vi "Clear Handle Map.vi"(8 "error in (no error)":errorcluster, 11 "TwinCAT ADS in":refnum<class "TwinCAT ADS.lvclass">) -> (0 "error out":errorcluster, 3 "TwinCAT ADS out":refnum<class "TwinCAT ADS.lvclass">)   [LabVIEW 2018, in "TwinCAT ADS.lvclass"]
uses:
  TwinCAT ADS.lvclass
  TwinCAT ADS.lvclass/TwinCAT ADS.ctl
panel:
  out "[Symbol Name]":string[](array[string])
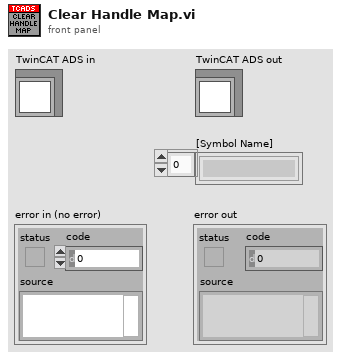
[diagram p1: front panel]
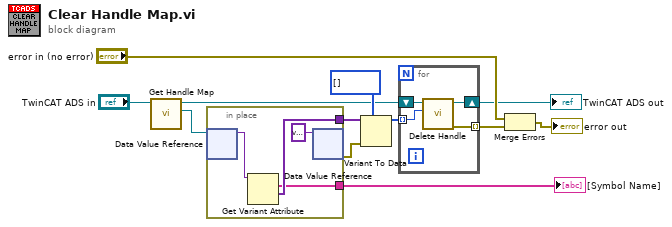
[diagram p0: block diagram]
diagram:
  n1 = call "Get Handle Map.vi"("TwinCAT ADS in"="TwinCAT ADS in") -> ("Handle Map"=w1:refnum<data-value>, "TwinCAT ADS out"=w2:refnum<class "TwinCAT ADS.lvclass">)  [unwired: 8 in, 1 out]
  n2 = in-place {
    in-place-border: [w14] -> w10
    in-place-border: [w13] -> w4
    n3 = in-place-dvr #1(w1) -> (w15:variant)  [unwired: 1 out]
    n4 = Get Variant Attribute(Variant=w15) -> (names=w13:string[], values=w14:variant[])  [unwired: 3 in, 2 out]
    n5 = in-place-dvr #1(variant ("data value")) -> (w11:errorcluster)  [unwired: 1 out]
  }
  "[Symbol Name]" <- w4
  n6 = Variant To Data(error in=w11, type=i32[] [], Variant=w10) -> (data=w8:i32[])  [unwired: 1 out]
  n7 = for {
    tunnel: w8 -> [w19] mode=indexing
    shift-right: [w17] -> w7
    shift-left: w2 -> [w20]
    tunnel: [w18] -> w6 mode=indexing
    n8 = call "Delete Handle.vi"("Handle"=w19, "TwinCAT ADS in"=w20) -> ("error out"=w18:errorcluster, "TwinCAT ADS out"=w17:refnum<class "TwinCAT ADS.lvclass">)  [unwired: 8 in]
  }
  "TwinCAT ADS out" <- w7
  n9 = Merge Errors("error in (no error)", w6) -> (→"error out":errorcluster)
